vi "host_restore.vi"() -> ()   [LabVIEW 2020]
uses:
  <vilib>/rvi/interface/RandomDataEmulation/nirviRandomDataOpen.vi
  <vilib>/rvi/interface/common/niFpgaCacheSessionInfoDynamic.vi
  <vilib>/Utility/error.llb/Error Cluster From Error Code.vi
  <vilib>/rvi/interface/common/niFpgaWaitOnOcc.vi
  <vilib>/rvi/errors/niLvFpgaAdjustHostInterfaceError.vi
  <vilib>/FPGAPlugInAG/Dynamic/niLvFpga_Run_Dynamic.vi
  <vilib>/FPGAPlugInAG/Dynamic/niLvFpga_Close_Dynamic.vi
  <vilib>/rvi/interface/nirviOpenFPGA/nirviOpenFPGA.xnode
  FFT.vi
  <vilib>/rvi/interface/nirviMethod/nirviMethod.xnode
  <vilib>/rvi/interface/nirviCloseFPGA/nirviCloseFPGA.xnode
  <vilib>/rvi/errors/niLvFpgaMergeErrorWithErrorCode.vi
  <vilib>/Analysis/NI_AALPro.lvlib
  <vilib>/FPGAPlugInAG/Dynamic/niLvFpga_ReadFifo_Dynamic.vi
  <vilib>/FPGAPlugInAG/Dynamic/niLvFpga_ConfigureFifo_Dynamic.vi
  <vilib>/FPGAPlugInAG/Dynamic/niLvFpga_StartFifo_Dynamic.vi
  <vilib>/FPGAPlugInAG/Dynamic/niLvFpga_WriteFifo_Dynamic.vi
panel:
  out "array faul":i32
  out "array faul":fxp<+/-,32,16>[](array[numeric])
  out "freq index":dbl[](array[numeric])
  out "phase 2 index":dbl[](graph)
  out "phase 2 size":i32
  out "mag 2 index":dbl[](graph)
  out "mag 2 size":i32
  out "phase 2":fxp<+/-,32,15>[](array[numeric])
  out "mag 2":fxp<+/-,32,15>[](array[numeric])
  out "frequency index":dbl[](graph)
  out "frequency size":i32
  out "freq":fxp<+/-,32,15>[](array[numeric])
  out "magnitude":dbl[](graph)
  out "phase":dbl[](graph)
  out "phase size":i32
  out "mag size":i32
  out "phase 3":fxp<+/-,32,15>[](array[numeric])
  out "magnitude 2":fxp<+/-,32,15>[](array[numeric])
  out "Actual Depth":u32
  out "host to target":u32
  out "signal_target_to_host_fixed size(s)":i32
  out "target to host 1":u32
  out "signal target to host":dbl[][](graph)
  out "signal_target_to_host_fixed":fxp<+/-,24,7>[](array[numeric])
  out "Array 2":fxp<+/-,24,7>[](array[numeric])
  out "detrend acc":dbl[](graph)
  out "samples":i32
  out "input signal":T1(graph)
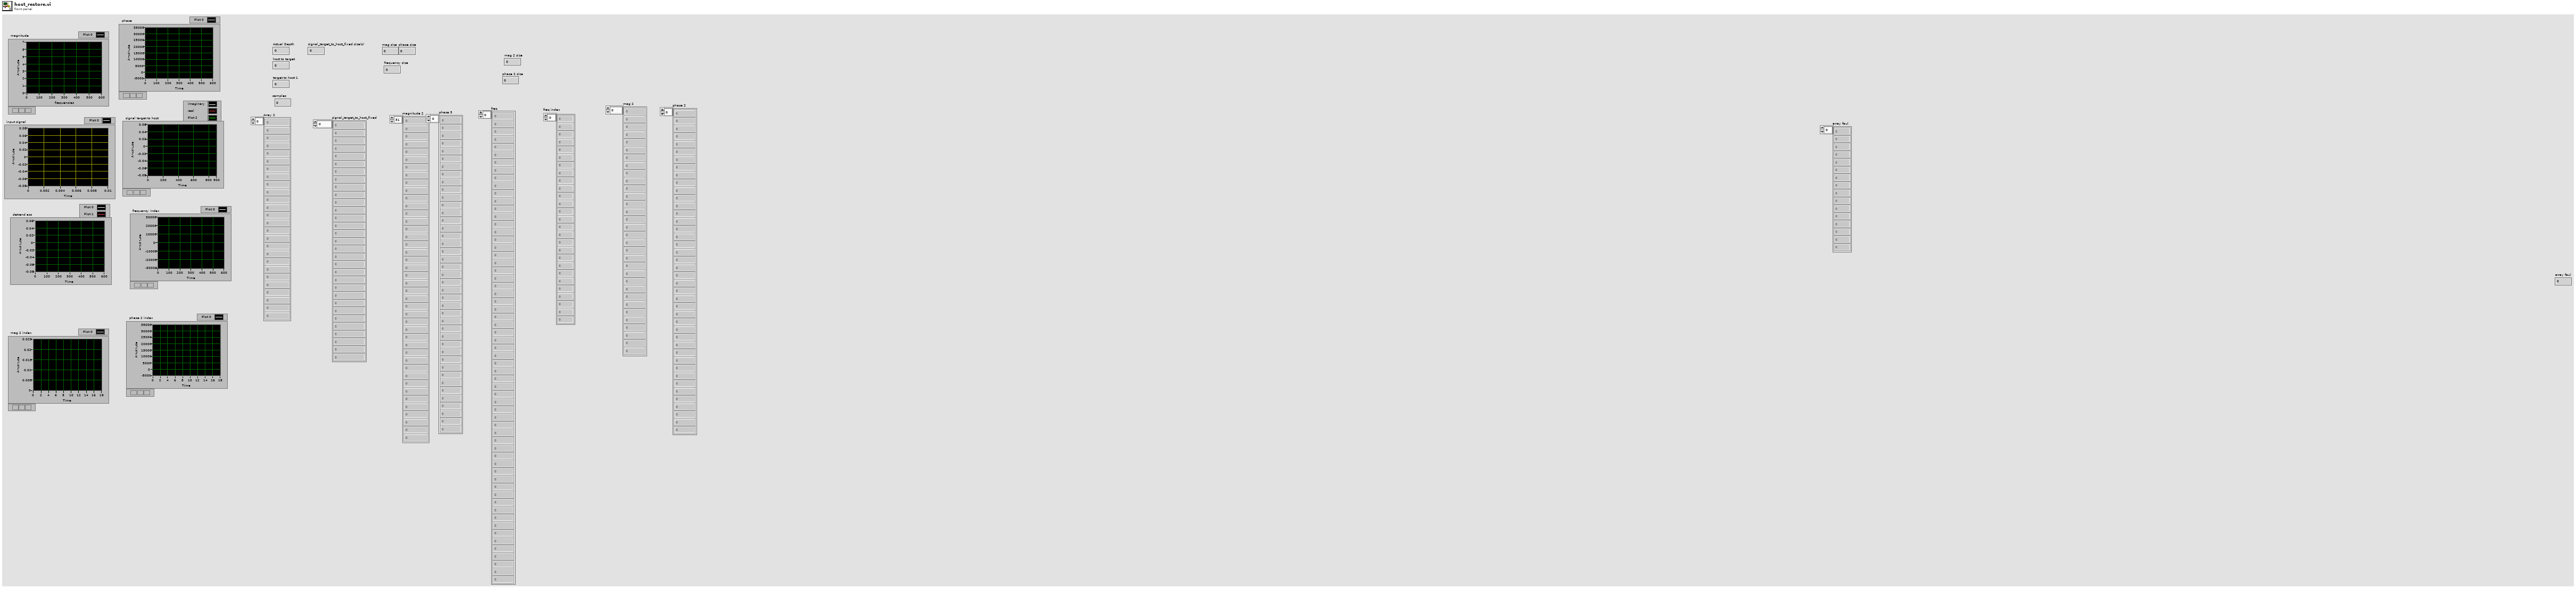
[diagram p1: front panel]
types:
  T1 = cluster{"array type (2D Dbl)":dbl[], "array type (2D Dbl)":dbl[]}
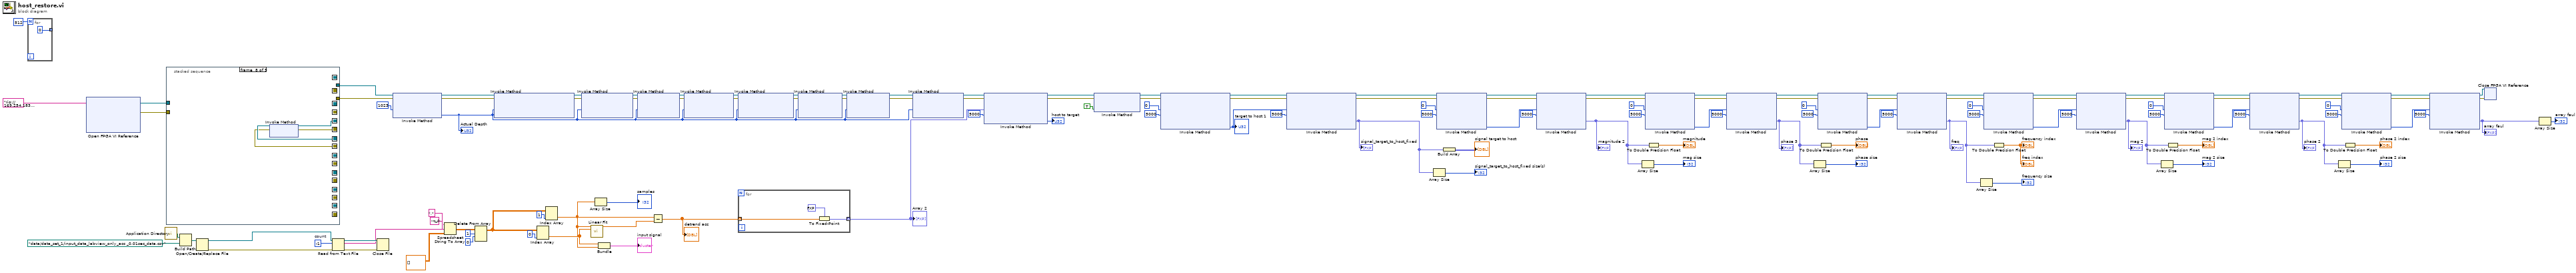
[diagram p0: block diagram]
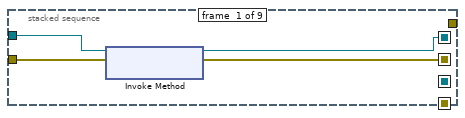
[diagram p2: hidden frame]
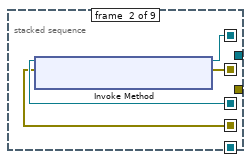
[diagram p3: hidden frame]
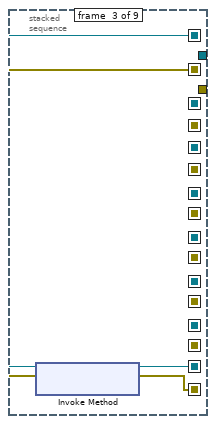
[diagram p4: hidden frame]
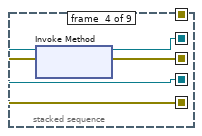
[diagram p5: hidden frame]
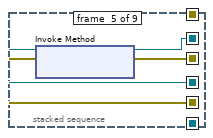
[diagram p6: hidden frame]
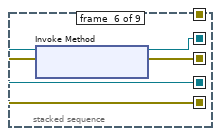
[diagram p7: hidden frame]
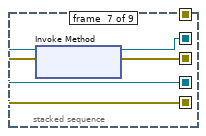
[diagram p8: hidden frame]
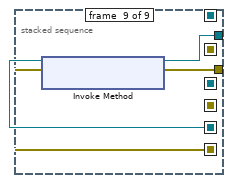
[diagram p9: hidden frame]
diagram:
  w125 = -1  # count
  n1 = for {
    N: 512 -> [_]
    tunnel: [0] -> _ mode=indexing
  }
  n2 = xnode "Open FPGA VI Reference"("resource name"=tag "rio://169.254.183.73/RIO0") -> ("FPGA VI Reference Out"=w95:refnum<k20>, "error out"=w94:errorcluster)  [unwired: 1 in]
  n3 = call <vilib>:"Application Directory.vi"() -> ("Application Directory"=w129:path)
  n4 = stacked-sequence {
    seq-local: [w137 _ _ _ _ _ _ _ _] -> [_ w143 _ _ _ _ _ _ _]
    seq-local: [w136 _ _ _ _ _ _ _ _] -> [_ w142 _ _ _ _ _ _ _]
    seq-local: [_ w141 _ _ _ _ _ _ _] -> [_ _ w147 _ _ _ _ _ _]
    seq-local: [_ w140 _ _ _ _ _ _ _] -> [_ _ w146 _ _ _ _ _ _]
    seq-local: [_ _ w145 _ _ _ _ _ _] -> [_ _ _ w151 _ _ _ _ _]
    seq-local: [_ _ w144 _ _ _ _ _ _] -> [_ _ _ w150 _ _ _ _ _]
    seq-local: [_ _ _ w149 _ _ _ _ _] -> [_ _ _ _ w155 _ _ _ _]
    seq-local: [_ _ _ w148 _ _ _ _ _] -> [_ _ _ _ w154 _ _ _ _]
    seq-local: [_ _ _ _ w153 _ _ _ _] -> [_ _ _ _ _ w159 _ _ _]
    seq-local: [_ _ _ _ w152 _ _ _ _] -> [_ _ _ _ _ w158 _ _ _]
    seq-local: [_ _ _ _ _ w157 _ _ _] -> [_ _ _ _ _ _ w163 _ _]
    seq-local: [_ _ _ _ _ w156 _ _ _] -> [_ _ _ _ _ _ w162 _ _]
    seq-local: [_ _ _ _ _ _ w161 _ _] -> [_ _ _ _ _ _ _ w166 _]
    seq-local: [_ _ _ _ _ _ w160 _ _] -> [_ _ _ _ _ _ _ w167 _]
    seq-local: [_ _ _ _ _ _ _ w165 _] -> [_ _ _ _ _ _ _ _ w171]
    seq-local: [_ _ _ _ _ _ _ w164 _] -> [_ _ _ _ _ _ _ _ w170]
    tunnel: w95 -> [w139 _ _ _ _ _ _ _ _]
    tunnel: w94 -> [w138 _ _ _ _ _ _ _ _]
    tunnel: [_ _ _ _ _ _ _ _ w169] -> w18
    tunnel: [_ _ _ _ _ _ _ _ w168] -> w17
    frame #0 {
      n5 = xnode "Invoke Method"("FPGA VI Reference In"=w139, "error in"=w138) -> ("FPGA VI Reference Out"=w137:refnum<k20>, "error out"=w136:errorcluster)
    }
    frame #1 {
      n6 = xnode "Invoke Method"("FPGA VI Reference In"=w143, "error in"=w142) -> ("FPGA VI Reference Out"=w141:refnum<k20>, "error out"=w140:errorcluster)
    }
    frame #2 {
      n7 = xnode "Invoke Method"("FPGA VI Reference In"=w147, "error in"=w146) -> ("FPGA VI Reference Out"=w145:refnum<k20>, "error out"=w144:errorcluster)
    }
    frame #3 {
      n8 = xnode "Invoke Method"("FPGA VI Reference In"=w151, "error in"=w150) -> ("FPGA VI Reference Out"=w149:refnum<k20>, "error out"=w148:errorcluster)
    }
    frame #4 {
      n9 = xnode "Invoke Method"("FPGA VI Reference In"=w155, "error in"=w154) -> ("FPGA VI Reference Out"=w153:refnum<k20>, "error out"=w152:errorcluster)
    }
    frame #5 {
      n10 = xnode "Invoke Method"("FPGA VI Reference In"=w159, "error in"=w158) -> ("FPGA VI Reference Out"=w157:refnum<k20>, "error out"=w156:errorcluster)
    }
    frame #6 {
      n11 = xnode "Invoke Method"("FPGA VI Reference In"=w163, "error in"=w162) -> ("FPGA VI Reference Out"=w160:refnum<k20>, "error out"=w161:errorcluster)
    }
    frame #7 {
      n12 = xnode "Invoke Method"("FPGA VI Reference In"=w167, "error in"=w166) -> ("FPGA VI Reference Out"=w165:refnum<k20>, "error out"=w164:errorcluster)
    }
    frame #8 {
      n13 = xnode "Invoke Method"("FPGA VI Reference In"=w171, "error in"=w170) -> ("FPGA VI Reference Out"=w169:refnum<k20>, "error out"=w168:errorcluster)
    }
  }
  n14 = Build Path(base path=w129, name or relative path=path "data/data_set_1/input_data_labview_only_acc _0.01sec_data.csv" ("default name")) -> (appended path=w128:path)
  n15 = Open/Create/Replace File(file path (use dialog)=w128) -> (refnum out=w133:refnum<file>, error out=w134:errorcluster)  [unwired: 5 in, 1 out]
  n16 = Read from Text File(file (use dialog)=w133, count=w125, error in=w134) -> (refnum out=w132:refnum<file>, text=w130:string, error out=w131:errorcluster)  [unwired: 1 in, 1 out]
  n17 = Close File(refnum=w132, error in=w131) -> ()  [unwired: 2 out]
  n18 = xnode "Invoke Method"("FPGA VI Reference In"=w18, "error in"=w17, "Requested Depth"=u32 1023) -> ("FPGA VI Reference Out"=w93:refnum<k20>, "error out"=w92:errorcluster, "Actual Depth"=w23:u32)
  "Actual Depth" <- w23
  n19 = Spreadsheet String To Array(delimiter (Tab)=",", format string="%f", spreadsheet string=w130, array type (2D Dbl)=dbl[][] []) -> (array=w122:dbl[][])
  n20 = Delete From Array(array=w122, length=1, index (row)=0) -> (array with subset deleted=w117:dbl[][])  [unwired: 1 in, 1 out]
  n21 = xnode "Invoke Method"("FPGA VI Reference In"=w93, "error in"=w92, "Requested Depth"=w23) -> ("FPGA VI Reference Out"=w91:refnum<k20>, "error out"=w90:errorcluster)  [unwired: 1 out]
  n22 = Index Array(array=w117, index (col)=0 ("disabled index (col)")) -> (element=w15:dbl[])  [unwired: 1 in]
  n23 = Index Array(array=w117, index (col)=1 ("disabled index (col)")) -> (element=w14:dbl[])  [unwired: 1 in]
  n24 = xnode "Invoke Method"("FPGA VI Reference In"=w91, "error in"=w90, "Requested Depth"=w23) -> ("FPGA VI Reference Out"=w89:refnum<k20>, "error out"=w88:errorcluster)  [unwired: 1 out]
  n25 = call <vilib>:"Linear Fit.vi"("Y"=w14, "X"=w15) -> ("Best Linear Fit"=w16:dbl[])  [unwired: 9 in, 4 out]
  n26 = Array Size(array=w14) -> (size(s)=→"samples":i32)
  n27 = Bundle("array type (2D Dbl)"=w15, "array type (2D Dbl)"=w14) -> (→"input signal":T1)  [unwired: 1 in]
  n28 = xnode "Invoke Method"("FPGA VI Reference In"=w89, "error in"=w88, "Requested Depth"=w23) -> ("FPGA VI Reference Out"=w55:refnum<k20>, "error out"=w54:errorcluster)  [unwired: 1 out]
  n29 = Subtract(x=w14, y=w16) -> (x-y=w109:dbl[])
  "detrend acc" <- w109
  n30 = xnode "Invoke Method"("FPGA VI Reference In"=w55, "error in"=w54, "Requested Depth"=w23) -> ("FPGA VI Reference Out"=w31:refnum<k20>, "error out"=w30:errorcluster)  [unwired: 1 out]
  n31 = xnode "Invoke Method"("FPGA VI Reference In"=w31, "error in"=w30, "Requested Depth"=w23) -> ("FPGA VI Reference Out"=w33:refnum<k20>, "error out"=w32:errorcluster)  [unwired: 1 out]
  n32 = for {
    tunnel: [w173] -> w108 mode=indexing
    tunnel: w109 -> [w172] mode=indexing
    n33 = To Fixed-Point(fixed-point type=fxp<+/-,24,7> 0.0 ("f"), number=w172) -> (fixed-point=w173:fxp<+/-,24,7>)
  }
  "Array 2" <- w108
  n34 = xnode "Invoke Method"("FPGA VI Reference In"=w33, "error in"=w32, "Requested Depth"=w23) -> ("FPGA VI Reference Out"=w25:refnum<k20>, "error out"=w24:errorcluster)  [unwired: 1 out]
  n35 = xnode "Invoke Method"("FPGA VI Reference In"=w25, "error in"=w24, "Requested Depth"=w23) -> ("FPGA VI Reference Out"=w22:refnum<k20>, "error out"=w21:errorcluster)  [unwired: 1 out]
  n36 = xnode "Invoke Method"("FPGA VI Reference In"=w22, "error in"=w21, "Requested Depth"=w23) -> ("FPGA VI Reference Out"=w20:refnum<k20>, "error out"=w19:errorcluster)  [unwired: 1 out]
  n37 = xnode "Invoke Method"("FPGA VI Reference In"=w20, "error in"=w19, "Data"=w108, "Timeout (ms)"=5000) -> ("FPGA VI Reference Out"=w114:refnum<k20>, "error out"=w113:errorcluster, "Empty Elements Remaining"=→"host to target":u32)
  n38 = xnode "Invoke Method"("FPGA VI Reference In"=w114, "error in"=w113, "Wait Until Done (F)"=TRUE) -> ("FPGA VI Reference Out"=w99:refnum<k20>, "error out"=w98:errorcluster)
  n39 = xnode "Invoke Method"("FPGA VI Reference In"=w99, "error in"=w98, "Number of Elements"=u32 0, "Timeout (ms)"=5000) -> ("FPGA VI Reference Out"=w107:refnum<k20>, "error out"=w106:errorcluster, "Elements Remaining"=w105:u32)  [unwired: 1 out]
  "target to host 1" <- w105
  n40 = xnode "Invoke Method"("FPGA VI Reference In"=w107, "error in"=w106, "Number of Elements"=w105, "Timeout (ms)"=5000) -> ("FPGA VI Reference Out"=w70:refnum<k20>, "error out"=w69:errorcluster, "Data"=w101:fxp<+/-,24,7>[])  [unwired: 1 out]
  "signal_target_to_host_fixed" <- w101
  n41 = Array Size(array=w101) -> (size(s)=→"signal_target_to_host_fixed size(s)":i32)
  n42 = xnode "Invoke Method"("FPGA VI Reference In"=w70, "error in"=w69, "Number of Elements"=u32 0, "Timeout (ms)"=5000) -> ("FPGA VI Reference Out"=w84:refnum<k20>, "error out"=w83:errorcluster, "Elements Remaining"=w78:u32)  [unwired: 1 out]
  n43 = Build Array(w101) -> (→"signal target to host":fxp<+/-,24,7>[][])
  n44 = xnode "Invoke Method"("FPGA VI Reference In"=w84, "error in"=w83, "Number of Elements"=w78, "Timeout (ms)"=5000) -> ("FPGA VI Reference Out"=w82:refnum<k20>, "error out"=w81:errorcluster, "Data"=w68:fxp<+/-,32,16>[])  [unwired: 1 out]
  "magnitude 2" <- w68
  n45 = Array Size(array=w68) -> (size(s)=→"mag size":i32)
  n46 = xnode "Invoke Method"("FPGA VI Reference In"=w82, "error in"=w81, "Number of Elements"=u32 0, "Timeout (ms)"=5000) -> ("FPGA VI Reference Out"=w80:refnum<k20>, "error out"=w79:errorcluster, "Elements Remaining"=w74:u32)  [unwired: 1 out]
  n47 = To Double Precision Float(number=w68) -> (double precision float=→"magnitude":dbl[])
  n48 = xnode "Invoke Method"("FPGA VI Reference In"=w80, "error in"=w79, "Number of Elements"=w74, "Timeout (ms)"=5000) -> ("FPGA VI Reference Out"=w57:refnum<k20>, "error out"=w56:errorcluster, "Data"=w67:fxp<+/-,32,16>[])  [unwired: 1 out]
  "phase 3" <- w67
  n49 = Array Size(array=w67) -> (size(s)=→"phase size":i32)
  n50 = xnode "Invoke Method"("FPGA VI Reference In"=w57, "error in"=w56, "Number of Elements"=u32 0, "Timeout (ms)"=5000) -> ("FPGA VI Reference Out"=w66:refnum<k20>, "error out"=w65:errorcluster, "Elements Remaining"=w62:u32)  [unwired: 1 out]
  n51 = To Double Precision Float(number=w67) -> (double precision float=→"phase":dbl[])
  n52 = xnode "Invoke Method"("FPGA VI Reference In"=w66, "error in"=w65, "Number of Elements"=w62, "Timeout (ms)"=5000) -> ("FPGA VI Reference Out"=w41:refnum<k20>, "error out"=w40:errorcluster, "Data"=w59:fxp<+/-,32,16>[])  [unwired: 1 out]
  "freq" <- w59
  n53 = Array Size(array=w59) -> (size(s)=→"frequency size":i32)
  n54 = xnode "Invoke Method"("FPGA VI Reference In"=w41, "error in"=w40, "Number of Elements"=u32 0, "Timeout (ms)"=5000) -> ("FPGA VI Reference Out"=w53:refnum<k20>, "error out"=w52:errorcluster, "Elements Remaining"=w49:u32)  [unwired: 1 out]
  n55 = To Double Precision Float(number=w59) -> (double precision float=→"frequency index" →"freq index":dbl[])
  n56 = xnode "Invoke Method"("FPGA VI Reference In"=w53, "error in"=w52, "Number of Elements"=w49, "Timeout (ms)"=5000) -> ("FPGA VI Reference Out"=w39:refnum<k20>, "error out"=w38:errorcluster, "Data"=w35:fxp<+/-,32,16>[])  [unwired: 1 out]
  "mag 2" <- w35
  n57 = Array Size(array=w35) -> (size(s)=→"mag 2 size":i32)
  n58 = xnode "Invoke Method"("FPGA VI Reference In"=w39, "error in"=w38, "Number of Elements"=u32 0, "Timeout (ms)"=5000) -> ("FPGA VI Reference Out"=w47:refnum<k20>, "error out"=w46:errorcluster, "Elements Remaining"=w43:u32)  [unwired: 1 out]
  n59 = To Double Precision Float(number=w35) -> (double precision float=→"mag 2 index":dbl[])
  n60 = xnode "Invoke Method"("FPGA VI Reference In"=w47, "error in"=w46, "Number of Elements"=w43, "Timeout (ms)"=5000) -> ("FPGA VI Reference Out"=w6:refnum<k20>, "error out"=w5:errorcluster, "Data"=w34:fxp<+/-,32,16>[])  [unwired: 1 out]
  "phase 2" <- w34
  n61 = Array Size(array=w34) -> (size(s)=→"phase 2 size":i32)
  n62 = xnode "Invoke Method"("FPGA VI Reference In"=w6, "error in"=w5, "Number of Elements"=u32 0, "Timeout (ms)"=5000) -> ("FPGA VI Reference Out"=w12:refnum<k20>, "error out"=w11:errorcluster, "Elements Remaining"=w8:u32)  [unwired: 1 out]
  n63 = To Double Precision Float(number=w34) -> (double precision float=→"phase 2 index":dbl[])
  n64 = xnode "Invoke Method"("FPGA VI Reference In"=w12, "error in"=w11, "Number of Elements"=w8, "Timeout (ms)"=5000) -> ("FPGA VI Reference Out"=w4:refnum<k20>, "error out"=w3:errorcluster, "Data"=w1:fxp<+/-,33,17>[])  [unwired: 1 out]
  "array faul" <- w1
  n65 = xnode "Close FPGA VI Reference"("FPGA VI Reference In"=w4, "error in"=w3) -> ()  [unwired: 1 out]
  n66 = Array Size(array=w1) -> (size(s)=→"array faul":i32)
